vi "SVN Checkout.vi"(8 "error in (no error)":errorcluster, 10 "ADT version":i32) -> (0 "error out":errorcluster, 1 "Successful Checkout":bool, 2 "Revision":i32, 3 "standard output":string)   [LabVIEW 2012, in "Design Server.lvlib"]
uses:
  Design Server.lvlib
  ReadWrite.ctl
  Folders.ctl
panel:
  out "standard error":string
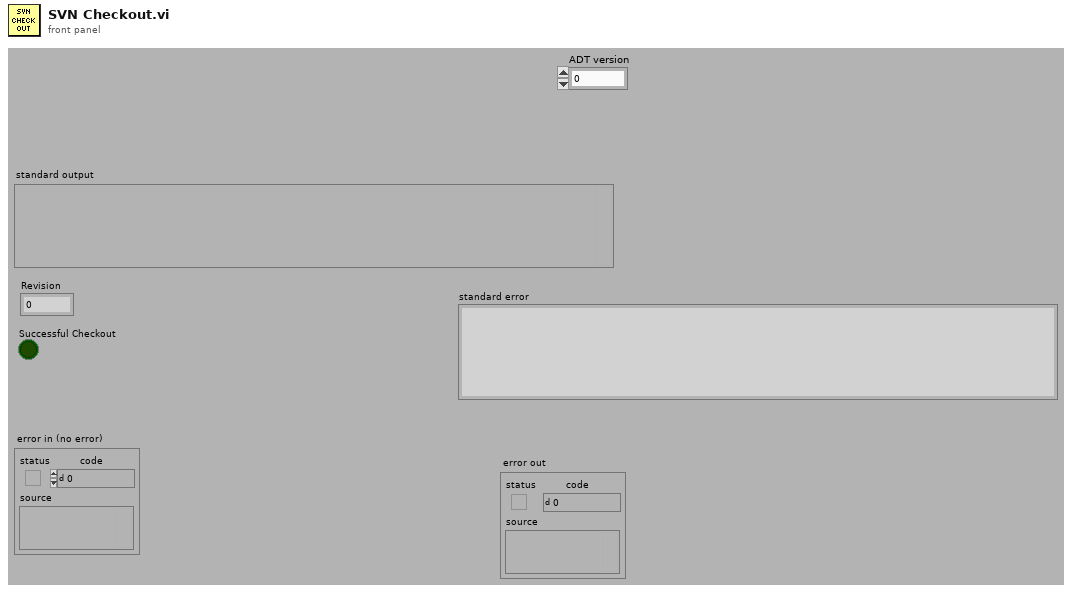
[diagram p1: front panel]
types:
  T1 = typedef "Design Server.lvlib/Folders.ctl" = enum16{"MathcadMethods", "RequestedDesigns", "CompletedDesigns", "MathcadCode", "CollabnetSVN.exe"}
  T2 = typedef "ReadWrite.ctl" = enum16{"Read", "Write"}
  T3 = typedef "SVN.ctl" = cluster{"Mathcad Code Repository":string, "Username":string, "Password":string, "Method file names (w extension)":string}
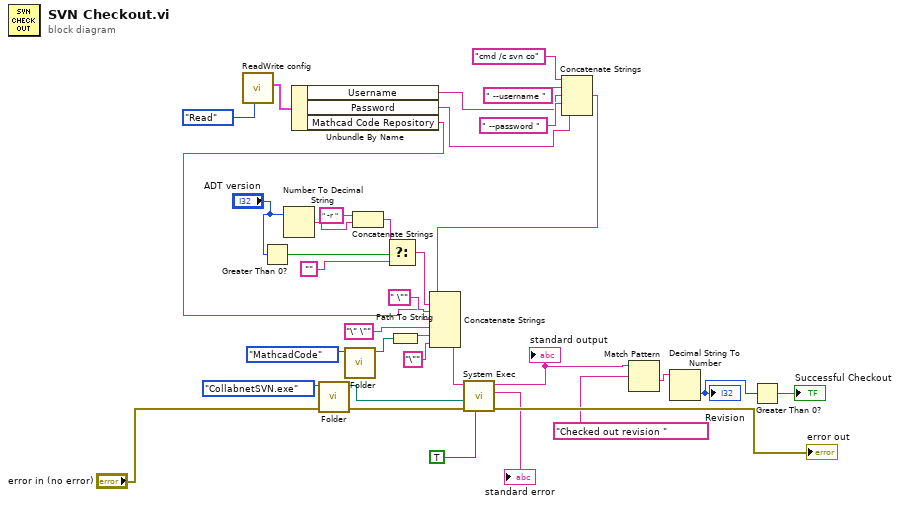
[diagram p0: block diagram]
diagram:
  n1 = call "ReadWrite config.vi"("Config"=ReadWrite."Read") -> ("SVN"=w13:T3)  [unwired: 7 in, 3 out]
  n2 = Greater Than 0?(x="ADT version") -> (x > 0?=w20:bool)
  n3 = Number To Decimal String(number="ADT version") -> (decimal integer string=w16:string)  [unwired: 1 in]
  n4 = Unbundle By Name(w13) -> ("Username"=w10:string, "Password"=w12:string, "Mathcad Code Repository"=w5:string)
  n5 = call "Folder.vi"("Folders"=Folders."CollabnetSVN.exe") -> ("FolderPath"=w3:path)  [unwired: 8 in, 2 out]
  n6 = call "Folder.vi"("Folders"=Folders."MathcadCode") -> ("FolderPath"=w1:path)  [unwired: 8 in, 2 out]
  n7 = Concatenate Strings(" -r " ("string"), w16) -> (w18:string)
  n8 = Select(t=w18, s=w20, f="") -> (s? t:f=w15:string)
  n9 = Path To String(path=w1) -> (string=w31:string)
  n10 = Concatenate Strings("cmd /c svn co" ("command"), " --username " ("string"), w10, " --password " ("string"), w12) -> (w6:string)
  n11 = Concatenate Strings(w6, w15, " \"" ("string"), w5, "\" \"" ("string"), w31, "\"" ("string")) -> (w30:string)
  n12 = call <vilib>:"System Exec.vi"("run minimized? (F)"=TRUE, "error in (no error)"="error in (no error)", "working directory"=w3, "command line"=w30) -> ("error out"=→"error out":errorcluster, "standard error"=→"standard error":string, "standard output"=w26:string)  [unwired: 4 in, 1 out]
  "standard output" <- w26
  n13 = Match Pattern(string=w26, regular expression="Checked out revision ") -> (after substring=w24:string)  [unwired: 1 in, 3 out]
  n14 = Decimal String To Number(string=w24) -> (number=w23:i32)  [unwired: 2 in, 1 out]
  "Revision" <- w23
  n15 = Greater Than 0?(x=w23) -> (x > 0?=→"Successful Checkout":bool)
